vi "Lang Set Frame Basic.vi"(8 "error in (no error)":errorcluster, 9 "Frame Skill":T1, 10 "Frame Basic":T3, 11 "LF2R IDE in":refnum<class "Main Panel.lvclass">) -> (0 "error out":errorcluster, 3 "LF2R IDE out":refnum<class "Main Panel.lvclass">)   [LabVIEW 2018, in "Main Panel.lvlib" / "Main Panel.lvclass"]
uses:
  Main Panel.lvclass
  Framework/Framework/Const Lang MainWnd Frame Basic.ctl
  Framework/Framework/Const Lang Property.ctl
  Framework/Framework/Const Lang MainWnd Frame Skill.ctl
  Main Panel.lvclass/Main Panel.ctl
  Framework/Framework/Framework.lvclass
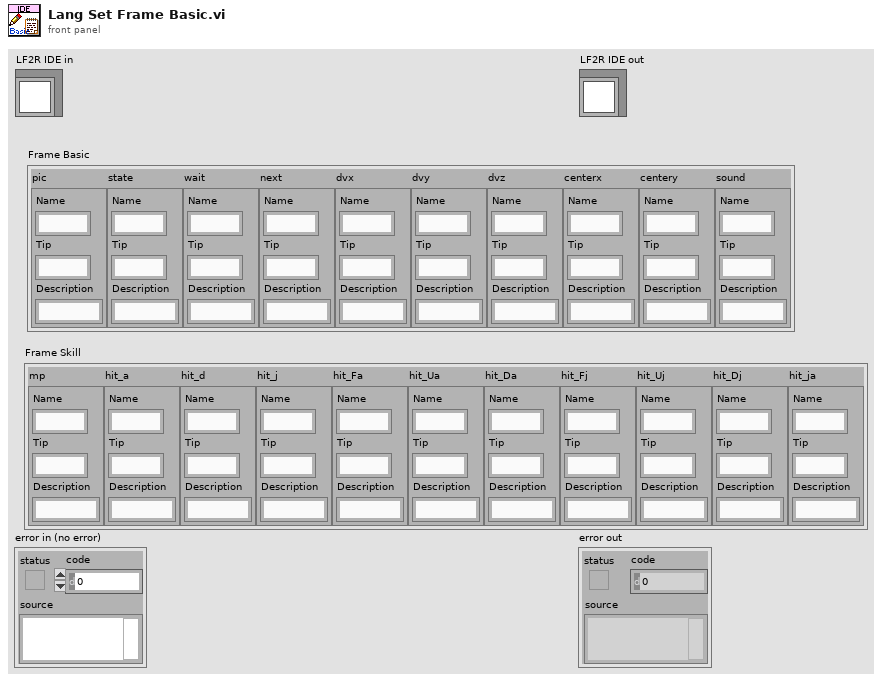
[diagram p1: front panel]
types:
  T1 = typedef "Framework.lvlib/Framework.lvclass/Const Lang MainWnd Frame Skill.ctl" = cluster{"mp":T2, "hit_a":T2, "hit_d":T2, "hit_j":T2, "hit_Fa":T2, "hit_Ua":T2, "hit_Da":T2, "hit_Fj":T2, "hit_Uj":T2, "hit_Dj":T2, "hit_ja":T2}
  T2 = typedef "Framework.lvlib/Framework.lvclass/Const Lang Property.ctl" = cluster{"Name":string, "Tip":string, "Description":string}
  T3 = typedef "Framework.lvlib/Framework.lvclass/Const Lang MainWnd Frame Basic.ctl" = cluster{"pic":T2, "state":T2, "wait":T2, "next":T2, "dvx":T2, "dvy":T2, "dvz":T2, "centerx":T2, "centery":T2, "sound":T2}
  T4 = cluster{"dvx":refnum<vi>, "dvy":refnum<vi>, "dvz":refnum<vi>}
  T5 = cluster{"centerx":refnum<vi>, "centery":refnum<vi>}
  T6 = cluster{"hit_a":refnum<vi>, "hit_d":refnum<vi>, "hit_j":refnum<vi>, "hit_Fa":refnum<vi>, "hit_Ua":refnum<vi>, "hit_Da":refnum<vi>, "hit_Fj":refnum<vi>, "hit_Uj":refnum<vi>, "hit_Dj":refnum<vi>, "hit_ja":refnum<vi>}
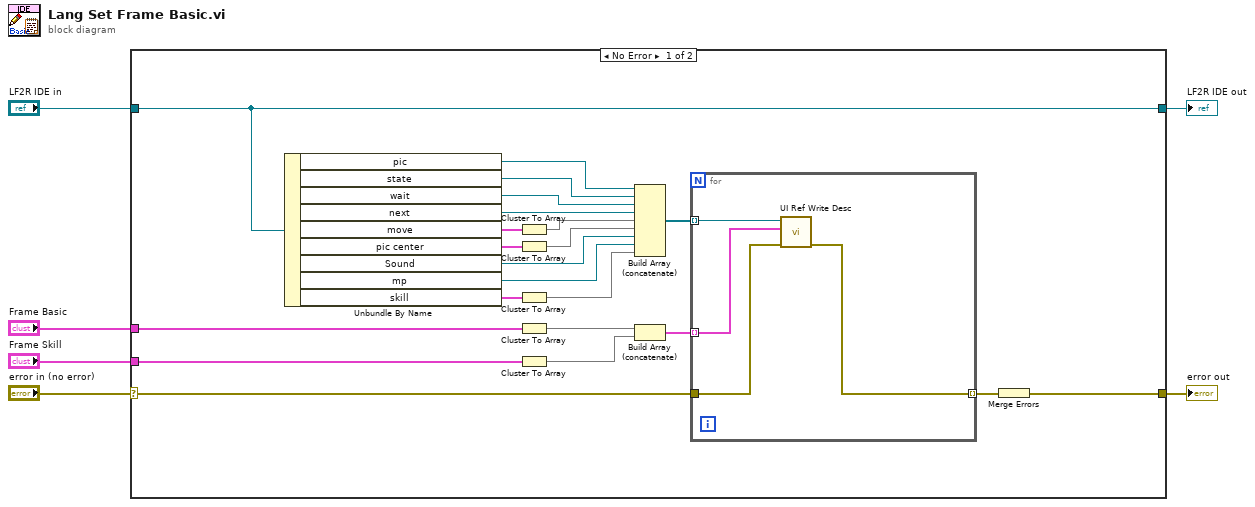
[diagram p0: block diagram]
diagram:
  n1 = case shown="No Error" "error in (no error)" {
    selector: "error in (no error)" -> [w14 w34]
    tunnel: [w12 w34] -> w5
    tunnel: [w28 w33] -> w3
    tunnel: "LF2R IDE in" -> [w28 w33]
    tunnel: "Frame Basic" -> [w19 _]
    tunnel: "Frame Skill" -> [w18 _]
    frame No Error {
      n2 = Unbundle By Name(w28) -> ("pic"=w10:refnum<vi>, "state"=w9:refnum<vi>, "wait"=w8:refnum<vi>, "next"=w7:refnum<vi>, "move"=w27:T4, "pic center"=w25:T5, "Sound"=w11:refnum<vi>, "mp"=w22:refnum<vi>, "skill"=w26:T6)
      n3 = Cluster To Array(cluster=w27) -> (array=w24:refnum<vi>[])
      n4 = Cluster To Array(cluster=w25) -> (array=w23:refnum<vi>[])
      n5 = Cluster To Array(cluster=w26) -> (array=w21:refnum<vi>[])
      n6 = Cluster To Array(cluster=w19) -> (array=w17:T2[])
      n7 = Cluster To Array(cluster=w18) -> (array=w16:T2[])
      n8 = Build Array (concatenate)(w10, w9, w8, w7, w24, w23, w11, w22, w21) -> (w20:refnum<vi>[])
      n9 = Build Array (concatenate)(w17, w16) -> (w15:T2[])
      n10 = for {
        tunnel: w20 -> [w32] mode=indexing
        tunnel: w15 -> [w31] mode=indexing
        tunnel: w14 -> [w30]
        tunnel: [w29] -> w13 mode=indexing
        n11 = call "UI Ref Write Desc.vi"("error in (no error)"=w30, "UI Property"=w31, "UI Ref"=w32) -> ("error out"=w29:errorcluster)  [unwired: 8 in]
      }
      n12 = Merge Errors(w13) -> (w12:errorcluster)
    }
    frame Error {
    }
  }
  "error out" <- w5
  "LF2R IDE out" <- w3
